vi "Create UEs.vi"(11 "Dev Actor Panel in":refnum<class "Dev Actor Panel.lvclass">) -> (0 "error out":errorcluster, 3 "Dev Actor Panel out":refnum<class "Dev Actor Panel.lvclass">)   [LabVIEW 2021, in "Dev Actor Panel.lvclass"]
uses:
  Dev Actor Panel.lvclass
  Dev Actor Panel.lvclass/Dev Actor Panel.ctl
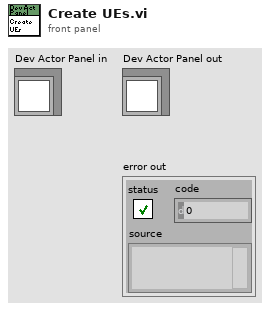
[diagram p1: front panel]
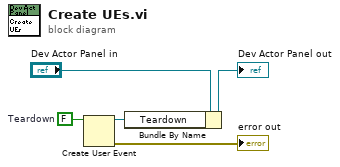
[diagram p0: block diagram]
diagram:
  w3 = FALSE  # Teardown
  n1 = Create User Event(user event datatype=w3) -> (user event=w2:refnum<user-event>, error out=→"error out":errorcluster)  [unwired: 1 in]
  n2 = Bundle By Name(cluster="Dev Actor Panel in", "Teardown"=w2) -> (→"Dev Actor Panel out":refnum<class "Dev Actor Panel.lvclass">)
